vi "Error merge.vi"(11 "Error details array":string[](array[string])) -> (3 "Detailed error out":string)   [LabVIEW 2015]
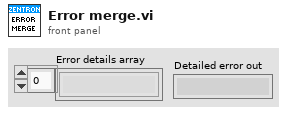
[diagram p1: front panel]
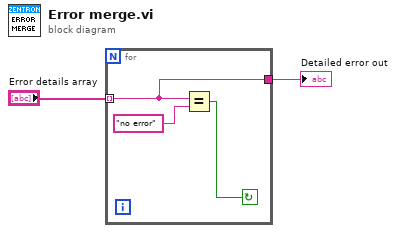
[diagram p0: block diagram]
diagram:
  n1 = for {
    tunnel: "Error details array" -> [w3] mode=indexing
    tunnel: [w3] -> w1
    stop <- w4 continue-if-true
    n2 = Equal?(x=w3, y="no error") -> (x = y?=w4:bool)
  }
  "Detailed error out" <- w1
